vi "test_logic.vi"() -> ()   [LabVIEW 2019]
panel:
  out "R6":bool
  out "R5":bool
  out "R4":bool
  out "R3":bool
  out "R2":bool
  out "R1":bool
  out "R8":bool
  out "R7":bool
  in  "input variable 2":dbl
  in  "input variable":dbl
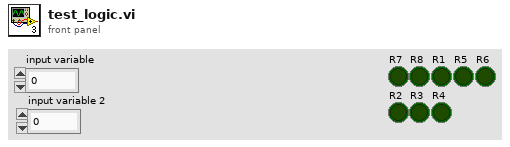
[diagram p1: front panel]
types:
  T1 = cluster{"Boolean array[0]":bool, "Boolean array[1]":bool, "Boolean array[2]":bool, "Boolean array[3]":bool, "Boolean array[4]":bool, "Boolean array[5]":bool, "Boolean array[6]":bool, "Boolean array[7]":bool}
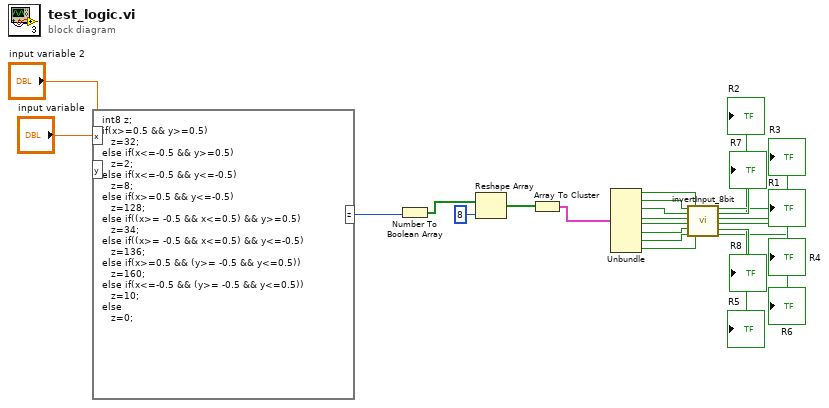
[diagram p0: block diagram]
diagram:
  n1 = formula code="int8 z;\nif(x>=0.5 && y>=0.5)\n   z=32;\nelse if(x<=-0.5 && y>=0.5)\n   z=2;\nelse if(x<=-0.5 && y<=-0.5)\n   z=8;\nelse if(x>=0.5 && y<=-0.5)\n   z=128;\nelse if((x>= -0.5 && x<=0.5) && y>=0.5)\n   z=34;\nelse if((x>= -0.5 && x<=0.5) && y<=-0.5)\n   z=136;\nelse if(x>=0.5 && (y>= -0.5 && y<=0.5))\n   z=160;\nelse if(x<=-0.5 && (y>= -0.5 && y<=0.5))\n   z=10;\nelse\n   z=0;"("x"="input variable", "y"="input variable 2") -> ("z"=w23:i8)
  n2 = Number To Boolean Array(number=w23) -> (Boolean array=w22:bool[])
  n3 = Reshape Array(w22, 8 ("dimension size")) -> (w20:bool[])
  n4 = Array To Cluster(array=w20) -> (cluster=w19:T1)
  n5 = Unbundle(w19) -> ("Boolean array[0]"=w18:bool, "Boolean array[1]"=w17:bool, "Boolean array[2]"=w16:bool, "Boolean array[3]"=w15:bool, "Boolean array[4]"=w14:bool, "Boolean array[5]"=w13:bool, "Boolean array[6]"=w12:bool, "Boolean array[7]"=w11:bool)
  n6 = call "invertInput_8bit.vi"("R2"=w17, "R3"=w16, "R4"=w15, "R5"=w14, "R6"=w13, "R7"=w12, "R1"=w18, "R8"=w11) -> ("R7"=→"R7":bool, "R8"=→"R8":bool, "R1"=→"R1":bool, "R2"=→"R2":bool, "R3"=→"R3":bool, "R4"=→"R4":bool, "R5"=→"R5":bool, "R6"=→"R6":bool)  [unwired: 4 in]
